vi "Final_keyboard (1).vi"() -> ()   [LabVIEW 2024]
uses:
  <vilib>/sound2/lvsound2.llb/Sampling Mode.ctl
  <vilib>/sound2/lvsound2.llb/Sound Data Format.ctl
  <vilib>/Instr/_visa.llb/VISA Configure Serial Port (Instr).vi
  <vilib>/Utility/inputDevices.llb/keyboardAcquire.vi
  <vilib>/Utility/inputDevices.llb/closeKeyboard.vi
  <vilib>/sound2/lvsound2.llb/Sound Output Set Volume (Single).vi
  <vilib>/sound2/lvsound2.llb/Sound Output Write (DBL Single).vi
  <vilib>/measure/NI_MABase.lvlib
panel:
  in  "Enum":T1(ring)
  out "Bufor odbiorczy":string
  in  "COM port set":refnum<visa-resource-name>
  in  "stop":bool
  out "Wygenerowany przebieg":waveform(dbl)(graph)
  in  "Regulacja głośności":dbl(knob) scale=0.0..100.0
  in  "oktawa":dbl min=-3.0 max=4.0 step=1.0
  out "Częstotliwość":dbl
  in  "Typ przebiegu":enum16{"Sine", "Square", "Triangle", "Sawtooth"}(ring)
  out "Indeks":u32
  in  "Klawisze pianina":T2(radio)=enum."C"
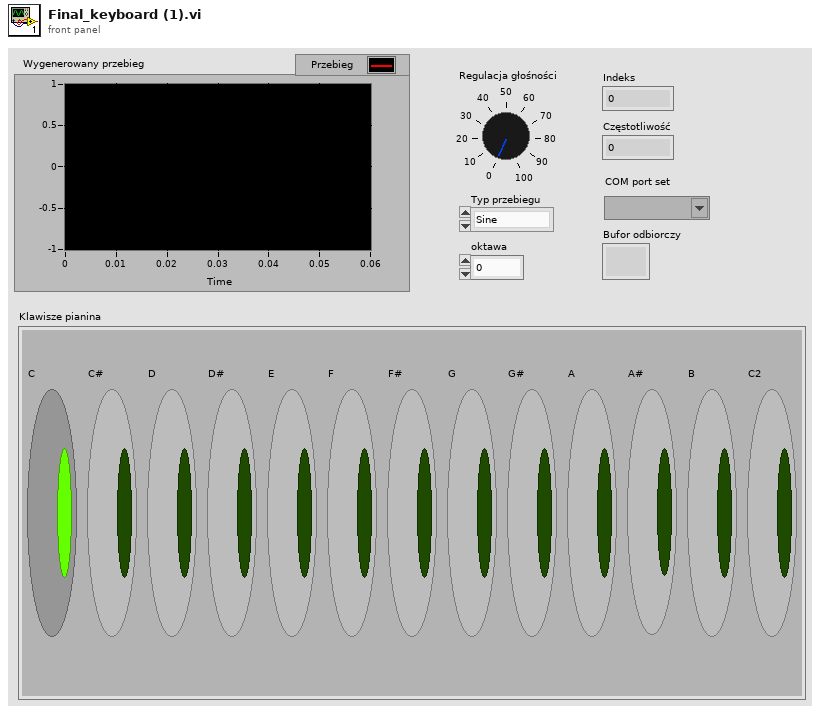
[diagram p1: front panel]
types:
  T1 = enum16{"No selection", "Boolean 1", "Boolean 2", "Boolean 3", "Boolean 4", "Boolean 5", "Boolean 6", "Boolean 7", "Boolean 8", "Boolean 9", "Boolean 10", "Boolean 11", "Boolean 12", "Boolean 13"}
  T2 = enum32{"No Selection", "C", "C#", "D", "D#", "E", "F", "F#", "G", "G#", "A", "A#", "B", "C2"}
  T3 = typedef "Sound Data Format.ctl" = cluster{"sample rate (S/s)":dbl, "number of channels":i32, "bits per sample":i32}
  T4 = typedef "Sampling Mode.ctl" = i32
  T5 = enum16{"0", "1", "2", "3", "4", "5", "6", "7", "8", "9", "A", "B", "C", "D", "E", "F", "G", "H", "I", "J", "K", "L", "M", "N", "O", "P", "Q", "R", "S", "T", "U", "V", "W", "X", "Y", "Z", "F1", "F2", "F3", "F4", "F5", "F6", "F7", "F8", "F9", "F10", "F11", "F12", "F13", "F14", "F15", "ADD", "BACK", "BACKSLASH", "CAPITAL", "COMMA", "DECIMAL", "DELETE", "DIVIDE", "DOWN", "END", "EQUALS", "ESCAPE", "GRAVE (`)", "HOME", "INSERT", "LBRACKET", "LCONTROL", "LEFT", "L ALT", "LSHIFT", "LWIN", "MINUS", "MULTIPLY", "NEXT", "NUMLOCK", "NUMPAD_0", "NUMPAD_1", "NUMPAD_2", "NUMPAD_3", "NUMPAD_4", "NUMPAD_5", "NUMPAD_6", "NUMPAD_7", "NUMPAD_8", "NUMPAD_9", "PAUSE", "PERIOD", "PRIOR (PG UP)", "RBRACKET", "RCONTROL", "RETURN", "RIGHT", "R ALT", "RSHIFT", "RWIN", "SCROLL", "SEMICOLON", "SLASH", "SPACE", "SUBTRACT", "TAB", "UP", "ENTER (num pad)", "' (quote)"}[]
  T6 = typedef "Sound Output Task ID.ctl" = u32
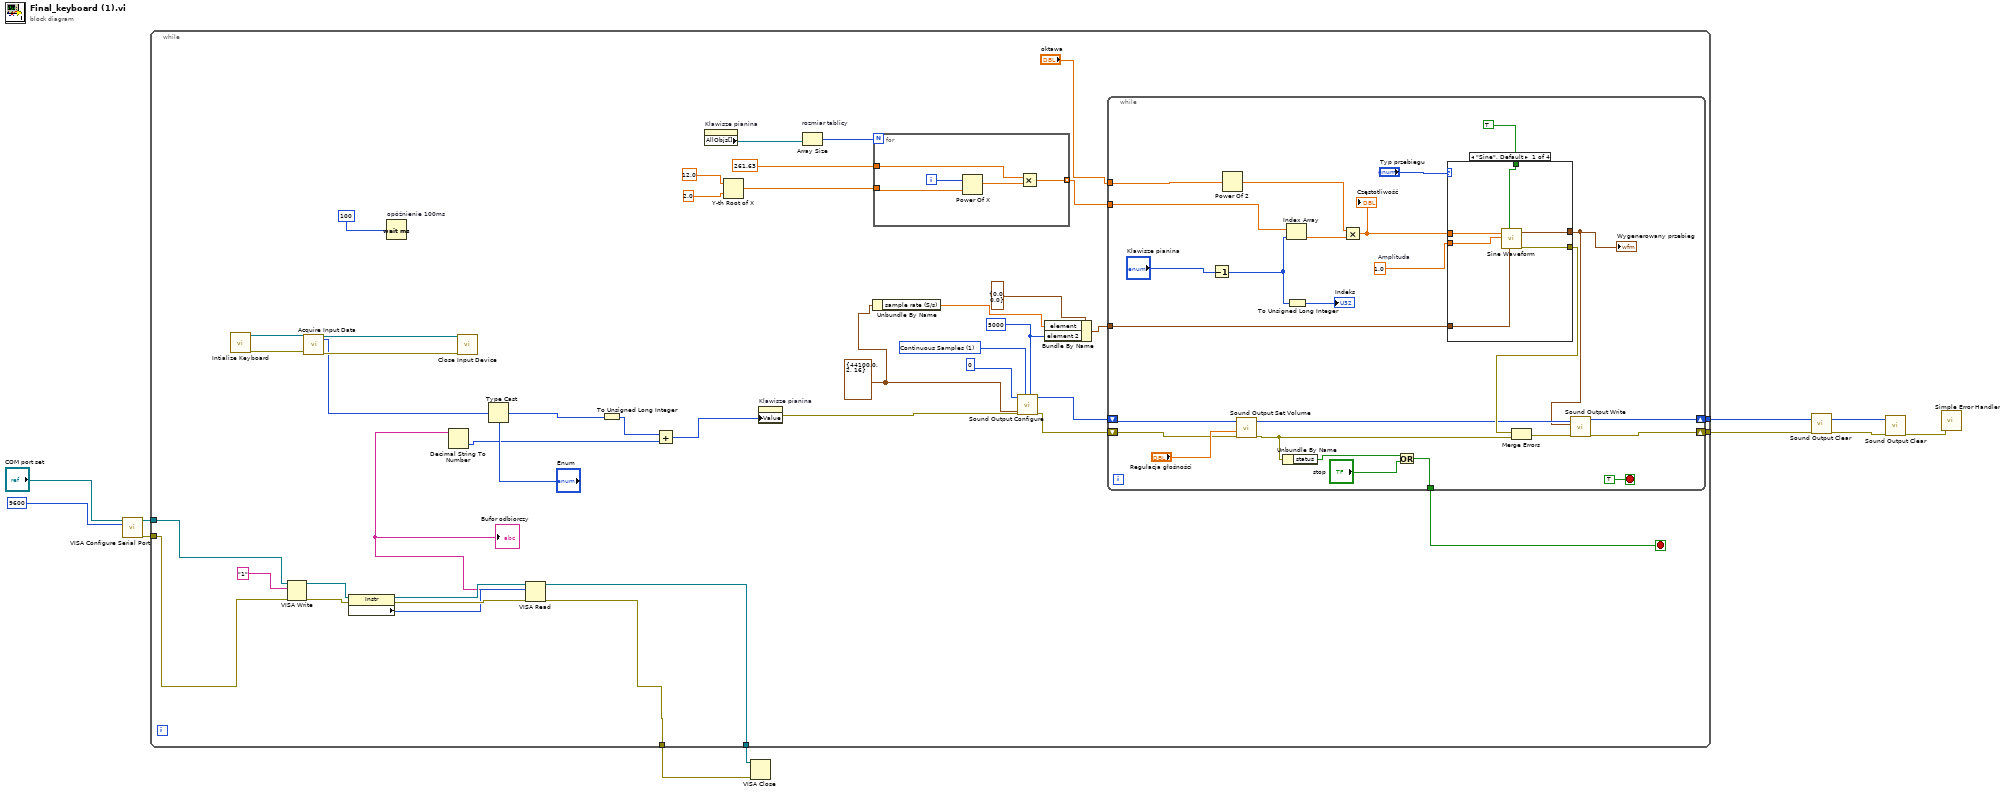
[diagram p0: block diagram]
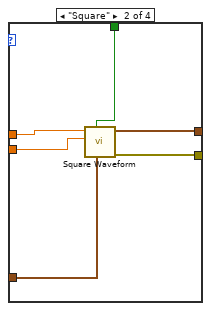
[diagram p2: hidden frame]
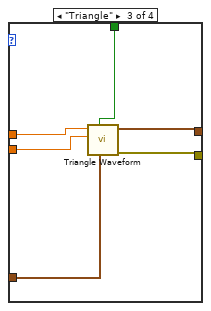
[diagram p3: hidden frame]
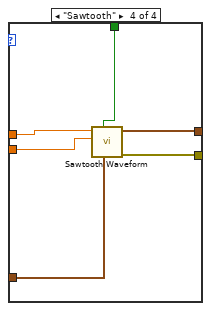
[diagram p4: hidden frame]
diagram:
  n1 = call-poly "VISA Configure Serial Port"("VISA resource name"="COM port set", "baud rate (9600)"=u32 9600) -> ("VISA resource name out"=w4:refnum<visa-resource-name>, "error out"=w3:errorcluster)  [unwired: 12 in]
  n2 = while {
    tunnel: [w42] -> w8
    tunnel: [w41] -> w9
    tunnel: w4 -> [w34]
    tunnel: w3 -> [w33]
    tunnel: [w32] -> w2
    tunnel: [w31] -> w1
    stop <- w40 stop-if-true
    w36 = T3 {"sample rate (S/s)"=44100.0, "number of channels"=2, "bits per sample"=16} ("sound format")
    w37 = 5000 ("number of samples/ch")
    w52 = T4 1 items=["Finite Samples", "Continuous Samples"] ("sample mode")
    n3 = call <vilib>:"Intialize Keyboard.vi"() -> ("error out"=w24:errorcluster, "device ID"=w25:refnum<k1>)  [unwired: 10 in]
    n4 = VISA Write(VISA resource name=w34, write buffer="1", error in (no error)=w33) -> (VISA resource name out=w29:refnum<visa-resource-name>, error out=w30:errorcluster)  [unwired: 1 out]
    n5 = call-poly <vilib>:"Acquire Input Data.vi"("device ID"=w25, "error in (no error)"=w24) -> ("device ID"=w22:refnum<k1>, "keys pressed"=w14:T5, "error out"=w23:errorcluster)  [unwired: 15 in]
    n6 = property class="Instr"(reference=w29, error in=w30) -> (reference out=w28:refnum<visa-resource-name>, error out=w27:errorcluster, "Serial Settings:Number of Bytes at Serial Port"=w26:u32)
    n7 = Wait (ms) "opóźnienie 100ms"(milliseconds to wait=u32 100) -> ()  [unwired: 1 out]
    n8 = call-poly <vilib>:"Close Input Device.vi"("error in (no error)"=w23, "device ID"=w22) -> ()  [unwired: 8 in, 1 out]
    n9 = Type Cast(type="Enum", x=w14) -> (*(type *) &x=w21:T1)
    n10 = VISA Read(VISA resource name=w28, byte count=w26, error in (no error)=w27) -> (VISA resource name out=w31:refnum<visa-resource-name>, read buffer=w15:string, error out=w32:errorcluster)  [unwired: 1 out]
    "Bufor odbiorczy" <- w15
    n11 = Decimal String To Number(string=w15) -> (number=w11:i32)  [unwired: 2 in, 1 out]
    n12 = To Unsigned Long Integer(number=w21) -> (unsigned 32bit integer=w13:u32)
    n13 = Add(x=w13, y=w11) -> (x+y=w12:u32)
    n14 = property on="Klawisze pianina" class="RadioBtnsControl (strict)"() -> ("AllObjs[]"=w50:refnum<vi>[])  [unwired: 2 in, 2 out]
    n15 = Y-th Root of X(1:2.0 ("y"), 2:12.0 ("x")) -> (0:w48:dbl)
    n16 = property on="Klawisze pianina" class="RadioBtnsControl (strict)"("Value"=w12) -> (error out=w17:errorcluster)  [unwired: 2 in, 1 out]
    n17 = Array Size "rozmiar tablicy"(array=w50) -> (size(s)=w49:i32)
    n18 = Unbundle By Name(w36) -> ("sample rate (S/s)"=w38:dbl)
    n19 = for {
      N: w49 -> [_]
      tunnel: 261.63 ("baza nut czy jaki chuj") -> [w56]
      tunnel: w48 -> [w55]
      tunnel: [w53] -> w45 mode=indexing
      i -> [w57]
      n20 = Power Of X(1:w55, 2:w57) -> (0:w54:dbl)
      n21 = Multiply(x=w56, y=w54) -> (x*y=w53:dbl)
    }
    n22 = call <vilib>:"Sound Output Configure.vi"("number of samples/ch"=w37, "sample mode"=w52, "error in (no error)"=w17, "sound format"=w36, "device ID"=u32 0) -> ("error out"=w44:errorcluster, "task ID"=w43:T6)  [unwired: 5 in]
    n23 = Bundle By Name(cluster=cluster{"element":dbl, "element 2":dbl} {"element"=0.0, "element 2"=0.0} ("input cluster"), "element"=w38, "element 2"=w37) -> (w35:cluster{"element":dbl, "element 2":dbl})
    n24 = while {
      tunnel: w35 -> [w78]
      tunnel: w45 -> [w77]
      tunnel: [w66] -> w40
      shift-right: [w73] -> w41
      shift-left: w44 -> [w75]
      shift-right: [w69] -> w42
      shift-left: w43 -> [w71]
      tunnel: "oktawa" -> [w62]
      stop <- TRUE stop-if-true
      w80 = 1.0  # Amplituda
      n25 = Decrement(x="Klawisze pianina") -> (x-1=w61:T2)
      n26 = Power Of 2 ("podnosi oktawę do kwadratu")(x=w62) -> (2^x=w81:dbl)
      n27 = call-poly <vilib>:"Sound Output Set Volume.vi"("error in (no error)"=w75, "volume"="Regulacja głośności", "task ID"=w71) -> ("error out"=w68:errorcluster, "task ID out"=w70:T6)  [unwired: 7 in]
      n28 = Unbundle By Name "Unbundle By Name"(w68) -> ("status"=w67:bool)
      n29 = Index Array ("Tablica indeksów-zwraca element tablicy o jakimś indeksie")(array=w77, index=w61) -> (element=w82:dbl)
      n30 = To Unsigned Long Integer ("konwertuje liczbe na 32- bitową liczbe całkowitą bez znaku")(number=w61) -> (unsigned 32bit integer=→"Indeks":u32)
      n31 = Multiply(x=w81, y=w82) -> (x*y=w79:dbl)
      "Częstotliwość" <- w79
      n32 = Or(x=w67, y="stop") -> (x .or. y?=w66:bool)
      n33 = case shown="\"Sine\", Default" "Typ przebiegu" {
        tunnel: w79 -> [w85 w94 w101 w107]
        tunnel: w80 -> [w86 w95 w100 w106]
        tunnel: [w89 w91 w97 w103] -> w65
        tunnel: [w88 w92 w98 w104] -> w72
        tunnel: w78 -> [w87 w93 w99 w105]
        tunnel: TRUE -> [w84 w90 w96 w102]
        frame "Sine", Default {
          n34 = call <vilib>:"Sine Waveform.vi"("sampling info"=w87, "reset signal"=w84, "amplitude"=w86, "frequency"=w85) -> ("error out"=w88:errorcluster, "signal out"=w89:waveform(dbl))  [unwired: 6 in]
        }
        frame "Square" {
          n35 = call <vilib>:"Square Waveform.vi"("sampling info"=w93, "reset signal"=w90, "amplitude"=w95, "frequency"=w94) -> ("error out"=w92:errorcluster, "signal out"=w91:waveform(dbl))  [unwired: 6 in]
        }
        frame "Triangle" {
          n36 = call <vilib>:"Triangle Waveform.vi"("sampling info"=w99, "reset signal"=w96, "amplitude"=w100, "frequency"=w101) -> ("error out"=w98:errorcluster, "signal out"=w97:waveform(dbl))  [unwired: 6 in]
        }
        frame "Sawtooth" {
          n37 = call <vilib>:"Sawtooth Waveform.vi"("sampling info"=w105, "reset signal"=w102, "amplitude"=w106, "frequency"=w107) -> ("error out"=w104:errorcluster, "signal out"=w103:waveform(dbl))  [unwired: 6 in]
        }
      }
      "Wygenerowany przebieg" <- w65
      n38 = Merge Errors(w72, w68) -> (w74:errorcluster)
      n39 = call-poly <vilib>:"Sound Output Write.vi"("error in (no error)"=w74, "data"=w65, "task ID"=w70) -> ("error out"=w73:errorcluster, "task ID out"=w69:T6)  [unwired: 7 in]
    }
  }
  n40 = VISA Close(VISA resource name=w1, error in (no error)=w2) -> ()  [unwired: 1 out]
  n41 = call <vilib>:"Sound Output Clear.vi"("error in (no error)"=w9, "task ID"=w8) -> ()  [unwired: 9 in, 1 out]
  n42 = call <vilib>:"Sound Output Clear.vi"("error in (no error)"=w9, "task ID"=w8) -> ("error out"=w7:errorcluster)  [unwired: 9 in]
  n43 = call <vilib>:"Simple Error Handler.vi"("error in (no error)"=w7) -> ()  [unwired: 4 in, 5 out]
